vi "Trial.vi"(0 "queue in":refnum<queue>, 5 "ADL":string="Pitcher", 11 "error in (no error)":errorcluster, 12 "motion (deg)":dbl=75.0 format="%#_13g", 13 "epsilon (deg)":dbl=5.0, 14 "hold (s)":dbl) -> (4 "queue out":refnum<queue>, 15 "error out":errorcluster)   [LabVIEW 2017]
uses:
  <vilib>/Analysis/8numeric.llb/1D Numeric Integration.vi
  <vilib>/Analysis/_algsub.llb/Real Vector Norm.vi
  <vilib>/Analysis/baseanly.llb/Outer Product.vi
  <vilib>/Analysis/baseanly.llb/Real Outer Product.vi
  <vilib>/robotics/Kinematics/Create Lie Group Matrix.vi
  Global.vi
  <vilib>/Analysis/7linalg.llb/Create Special Matrix.vi
  <vilib>/Analysis/7linalg.llb/Create Special Real Matrix.vi
  <vilib>/Analysis/Matrix/Numeric/Multiply/Multiply.vi
  <vilib>/Analysis/Matrix/Numeric/Multiply/Multiply - RM,R.vi
  <vilib>/Analysis/Matrix/Numeric/Multiply/Multiply - R,RM.vi
  <vilib>/Analysis/Matrix/Numeric/Add/Add.vi
  <vilib>/Analysis/Matrix/Numeric/Add/Add - RM,RM.vi
  <vilib>/Analysis/polynomials.llb/1D Polynomial Evaluation (DBL).vi
  Control/Damping.ctl
  <vilib>/robotics/Kinematics/NI_Kinematics.lvlib
  <vilib>/Analysis/NI_AALPro.lvlib
panel:
  out "P2P":dbl
  out "RMSE":dbl format="%0.4f"
  out "XY Graph":cluster{dbl[], dbl[]}[](graph)
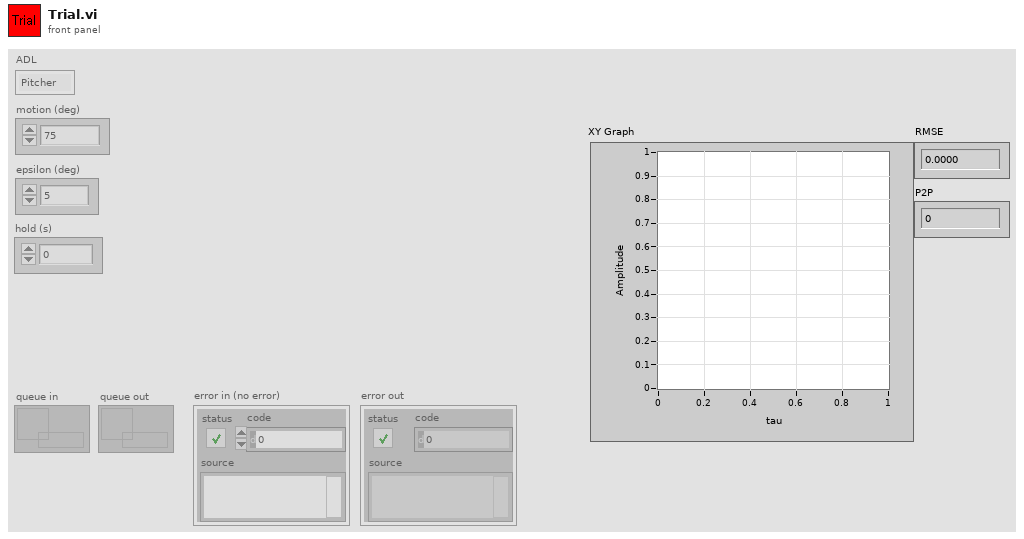
[diagram p1: front panel]
types:
  T1 = typedef "NI_Matrix.lvlib/RealMatrix.ctl" = dbl[][]
  T2 = typedef "Damping.ctl" = cluster{"bx":dbl, "by":dbl, "bz":dbl}
  T3 = typedef "Torque Vector.ctl" = cluster{"Tx":dbl, "Ty":dbl, "Tz":dbl}
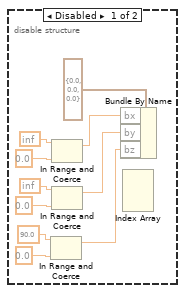
[diagram p2: hidden frame]
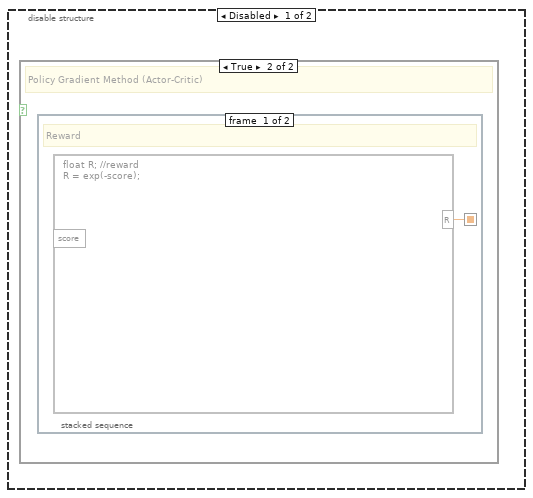
[diagram p3: hidden frame]
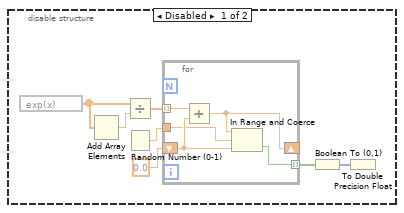
[diagram p6: hidden frame]
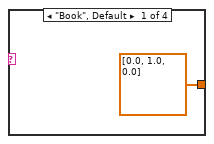
[diagram p7: hidden frame]
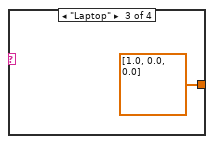
[diagram p8: hidden frame]
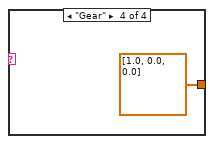
[diagram p9: hidden frame]
diagram:
  n1 = flat-sequence {
    tunnel: "queue in" -> [w17]
    tunnel: "error in (no error)" -> [w15]
    tunnel: [w14] -> w6
    tunnel: [w16] -> w5
    tunnel: "ADL" -> [w12]
    tunnel: "motion (deg)" -> [w11]
    tunnel: "epsilon (deg)" -> [w10]
    tunnel: "hold (s)" -> [w9]
    frame #0 {
      n2 = expression code="(x/180.0)*pi" "degrees to radians"(w11) -> (w13:dbl)
      n3 = case shown="\"Pitcher\"" w12 {
        tunnel: [dbl[] [0.0, 1.0, 0.0] dbl[] [0.0, -1.0, 0.0] dbl[] [1.0, 0.0, 0.0] dbl[] [1.0, 0.0, 0.0]] -> w18
        frame "Book", Default {
        }
        frame "Pitcher" {
        }
        frame "Laptop" {
        }
        frame "Gear" {
        }
      }
      n4 = while {
        tunnel: w13 -> [w31]
        tunnel: w18 -> [w55]
        tunnel: w10 -> [w54]
        shift-right: [w56] -> w16
        shift-left: w17 -> [w57]
        shift-right: [w39] -> w14
        shift-left: w15 -> [w42]
        tunnel: w9 -> [w26]
        i -> [w59]
        stop <- w58 stop-if-true
        w27 = u32 10 ("Trial Wait (ms)")
        n5 = Quotient & Remainder(x=w59, y=2) -> (x-y*floor(x/y)=w51:i32)  [unwired: 1 out]
        n6 = Equal To 0?(x=w51) -> (x = 0?=w37:bool)
        n7 = To Double Precision Float(number=w27) -> (double precision float=w28:dbl)
        n8 = Select(t=w31, s=w37, f=0.0) -> (s? t:f=w38:dbl)
        n9 = call <vilib>:"Angle Vector to Rotation Matrix.vi"("vector"=w55, "angle"=w38) -> ("rotation matrix"=w50:T1)
        n10 = Select(t="Forward" ("element"), s=w37, f="Backward" ("element")) -> (s? t:f=w47:string)
        n11 = global read "Global.vi" "EndEffector"() -> (w35:cluster{"roll":dbl, "pitch":dbl, "yaw":dbl})
        n12 = global read "Global.vi" "Damping"() -> (w24:T2)
        n13 = Obtain Queue(element data type="", error in (no error)=w42) -> (queue out=w53:refnum<queue>, error out=w46:errorcluster)  [unwired: 3 in, 1 out]
        n14 = Divide(x=w28, y=1000.0) -> (x/y=w25:dbl)
        n15 = Enqueue Element(queue=w57, element=w47, error in (no error)=w42) -> (queue out=w56:refnum<queue>, error out=w41:errorcluster)  [unwired: 1 in, 1 out]
        n16 = call <vilib>:"Rotation Matrix to Roll Pitch Yaw.vi"("rotation matrix"=w50) -> ("angles"=w33:cluster{"roll":dbl, "pitch":dbl, "yaw":dbl})
        n17 = global write "Global.vi" "Waypoint"(w33) -> ()
        n18 = Unbundle By Name(w33) -> ("pitch"=w32:dbl)
        n19 = Unbundle By Name(w35) -> ("pitch"=w34:dbl)
        n20 = Unbundle By Name(w24) -> ("by"=w23:dbl)
        n21 = flat-sequence {
          tunnel: w53 -> [w92]
          tunnel: w34 -> [w87]
          tunnel: w32 -> [w90]
          tunnel: w25 -> [w79]
          tunnel: w23 -> [w74]
          frame #0 {
            w88 = dbl[] [0.0, 0.0, 30.0, -60.0, 30.0, 0.0]  # MJT
            n22 = while {
              tunnel: w92 -> [w99]
              shift-right: [w98] -> w64
              shift-left: dbl[] [] -> [w97]
              stop <- w100 stop-if-true
              n23 = Dequeue Element(queue=w99) -> (error out=w96:errorcluster)  [unwired: 2 in, 3 out]
              n24 = case shown="No Error" w96 {
                tunnel: [w103 w105] -> w98
                tunnel: w97 -> [w102 w105]
                frame No Error {
                  n25 = global read "Global.vi" "Torque Vector"() -> (w104:T3)
                  n26 = Unbundle By Name(w104) -> ("Ty"=w101:dbl)
                  n27 = Build Array (concatenate)(w102, w101) -> (w103:dbl[])
                }
                frame Error {
                }
              }
              n28 = Unbundle By Name(w96) -> ("status"=w100:bool)
            }
            n29 = Subtract(x=w90, y=w87) -> (x-y=w78:dbl)
            n30 = Array Size(array=w64) -> (size(s)=w81:i32)
            n31 = To Double Precision Float(number=w81) -> (double precision float=w71:dbl)
            n32 = Multiply(x=w71, y=w79) -> (x*y=w77:dbl)
            n33 = for {
              N: w81 -> [_]
              shift-right: [w94] -> w89
              shift-left: i32[] [] -> [w93]
              i -> [w95]
              n34 = Build Array (concatenate)(w93, w95) -> (w94:i32[])
            }
            n35 = Divide(x=w78, y=w77) -> (x/y=w75:dbl)
            n36 = Reciprocal(x=w71) -> (1/x=w70:dbl)
            n37 = To Double Precision Float(number=w89) -> (double precision float=w82:dbl[])
            n38 = Divide(x=w82, y=w71) -> (x/y=w80:dbl[])
            n39 = call-poly <vilib>:"Polynomial Evaluation.vi"("P(x)"=w88, "A"=w80) -> ("P(A)"=w76:dbl[])  [unwired: 1 out]
            n40 = Compound Arithmetic op=MULTIPLY(w74, w75, w76) -> (w66:dbl[])
            n41 = Absolute Value(x=w66) -> (abs(x)=w67:dbl[])
            n42 = Array Max & Min(array=w67) -> (max value=w63:dbl)  [unwired: 3 out]
            n43 = Divide(x=w64, y=w63) -> (x/y=w61:dbl[])
            n44 = Divide(x=w66, y=w63) -> (x/y=w65:dbl[])
            n45 = Absolute Value(x=w61) -> (abs(x)=w62:dbl[])
            n46 = Subtract(x=w61, y=w65) -> (x-y=w73:dbl[])
            n47 = Bundle(w80, w61) -> (w86:cluster{dbl[], dbl[]})  [unwired: 1 in]
            n48 = Bundle(w80, w65) -> (w85:cluster{dbl[], dbl[]})  [unwired: 1 in]
            n49 = Array Max & Min(array=w62) -> (max value=→"P2P":dbl)  [unwired: 3 out]
            n50 = Square(x=w73) -> (x^2=w72:dbl[])
            n51 = Build Array(w86, w85) -> (→"XY Graph":cluster{dbl[], dbl[]}[])
            n52 = call-poly <vilib>:"Numeric Integration.vi"("dt"=w70, "Input Array"=w72) -> ("result"=w69:dbl)  [unwired: 1 in, 1 out]
            n53 = Square Root(x=w69) -> (sqrt(x)=→"RMSE":dbl)
          }
        }
        n54 = while {
          tunnel: w33 -> [w123]
          tunnel: w54 -> [w120]
          shift-right: [w118] -> w43
          shift-left: w46 -> [w119]
          shift-right: [w116] -> w44
          shift-left: w53 -> [w117]
          shift-right: [w108] -> _
          shift-left: 0.0 ("f") -> [w112]
          tunnel: w27 -> [w110]
          tunnel: w26 -> [w107]
          tunnel: w25 -> [w106]
          stop <- w128 stop-if-true
          # "Forward -> Backward -> Forward -> ..."
          n55 = Wait (ms)(milliseconds to wait=w110) -> ()  [unwired: 1 out]
          n56 = global read "Global.vi" "EndEffector"() -> (w122:cluster{"roll":dbl, "pitch":dbl, "yaw":dbl})
          n57 = global read "Global.vi" "Playback"() -> (w115:bool)
          n58 = Add(x=w112, y=w106) -> (x+y=w111:dbl)
          n59 = Subtract(x=w123, y=w122) -> (x-y=w121:cluster{"roll":dbl, "pitch":dbl, "yaw":dbl})
          n60 = case shown="True" w115 {
            tunnel: w119 -> [w129 w135]
            tunnel: [w129 w134] -> w118
            tunnel: w117 -> [w130 w133]
            tunnel: [w130 w132] -> w116
            frame False {
            }
            frame True {
              n61 = Enqueue Element(queue=w133, element="", error in (no error)=w135) -> (queue out=w132:refnum<queue>, error out=w134:errorcluster)  [unwired: 1 in, 1 out]
            }
          }
          n62 = expression code="(x/180.0)*pi" "degrees to radians"(w120) -> (w124:dbl)
          n63 = Cluster To Array(cluster=w121) -> (array=w126:dbl[])
          n64 = call-poly <vilib>:"Vector Norm.vi"("Input Vector"=w126) -> ("norm"=w125:dbl)  [unwired: 9 in, 1 out]
          n65 = Less?(x=w125, y=w124) -> (x < y?=w114:bool)
          n66 = Select(t=w111, s=w114, f=0.0) -> (s? t:f=w108:dbl)
          n67 = Greater?(x=w108, y=w107) -> (0:w109:bool)
          n68 = global read "Global.vi" "Stop"() -> (w127:bool)
          n69 = Or(x=w127, y=w109) -> (x .or. y?=w128:bool)
        }
        n70 = Release Queue(queue=w44, error in (no error)=w43) -> (error out=w40:errorcluster)  [unwired: 1 in, 2 out]
        n71 = Merge Errors(w40, w41) -> (w39:errorcluster)
        n72 = global read "Global.vi" "Stop"() -> (w58:bool)
      }
    }
  }
  n73 = disable-structure shown="Enabled" {
    frame Disabled {
      n74 = In Range and Coerce(upper limit=90.0, lower limit=0.0) -> (coerced(x)=w145:dbl)  [unwired: 1 in, 1 out]
      n75 = In Range and Coerce(upper limit=inf, lower limit=0.0) -> (coerced(x)=w143:dbl)  [unwired: 1 in, 1 out]
      n76 = In Range and Coerce(upper limit=inf, lower limit=0.0) -> (coerced(x)=w144:dbl)  [unwired: 1 in, 1 out]
      n77 = Bundle By Name(cluster=T2 {"bx"=0.0, "by"=0.0, "bz"=0.0} ("State"), "bx"=w143, "by"=w144, "bz"=w145) -> ()  [unwired: 1 out]
      n78 = Index Array() -> ()  [unwired: 4 in, 3 out]
    }
    frame Enabled {
    }
  }
  n79 = disable-structure shown="Enabled" {
    frame Disabled {
      n80 = expression code="exp(x)"() -> (w148:dbl[])  [unwired: 1 in]
      n81 = Add Array Elements(numeric array=w148) -> (sum=w149:dbl)
      n82 = Divide(x=w148, y=w149) -> (x/y=w146:dbl[])
      n83 = Random Number (0-1)() -> (number: 0 to 1=w150:dbl)
      n84 = for {
        shift-right: [w156] -> _
        shift-left: 0.0 -> [w157]
        tunnel: w150 -> [w155]
        tunnel: [w154] -> w151 mode=indexing
        tunnel: w146 -> [w153] mode=indexing
        n85 = Add(x=w153, y=w157) -> (x+y=w156:dbl)
        n86 = In Range and Coerce(upper limit=w156, x=w155, lower limit=w157) -> (In Range?=w154:bool)  [unwired: 1 out]
      }
      n87 = Boolean To (0,1)(Boolean=w151) -> (0, 1=w152:i16[])
      n88 = To Double Precision Float(number=w152) -> ()  [unwired: 1 out]
    }
    frame Enabled {
    }
  }
  n89 = disable-structure shown="Enabled" {
    frame Disabled {
      n90 = case shown="True" {
        selector: _ -> [_ _]
        frame False {
        }
        frame True {
          # "Policy Gradient Method (Actor-Critic)"
          n91 = stacked-sequence {
            seq-local: [w158 _] -> [_ _]
            frame #0 {
              # "Reward"
              n92 = formula code="float R; //reward\nR = exp(-score);"() -> ("R"=w158:dbl)  [unwired: 1 in]
            }
            frame #1 {
            }
          }
        }
      }
    }
    frame Enabled {
    }
  }
  "error out" <- w6
  "queue out" <- w5
